vi "CRH3605KitList.vi"() -> ()   [LabVIEW 2012]
uses:
  <vilib>/addons/database/Connection.llb/DB Tools Open Connec (Path).vi
  Global1.vi
  <vilib>/Utility/file.llb/Read From Spreadsheet File (string).vi
  <vilib>/addons/database/NI_Database_API.lvlib
panel:
  out "error out":errorcluster
  in  "Cluster":T1
  out "String":string
  out "date/time string":string
  out "path":path
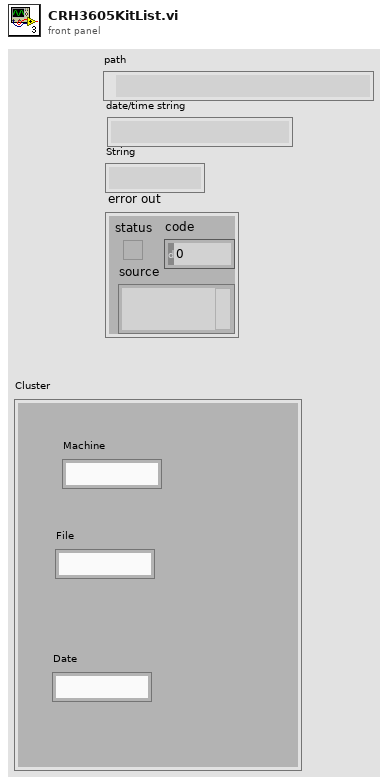
[diagram p1: front panel]
types:
  T1 = cluster{"Machine":string, "File":string, "Date":string}
  T2 = typedef "NI_Database_API.lvlib/Conn ObjectReference.ctl" = refnum<k1>
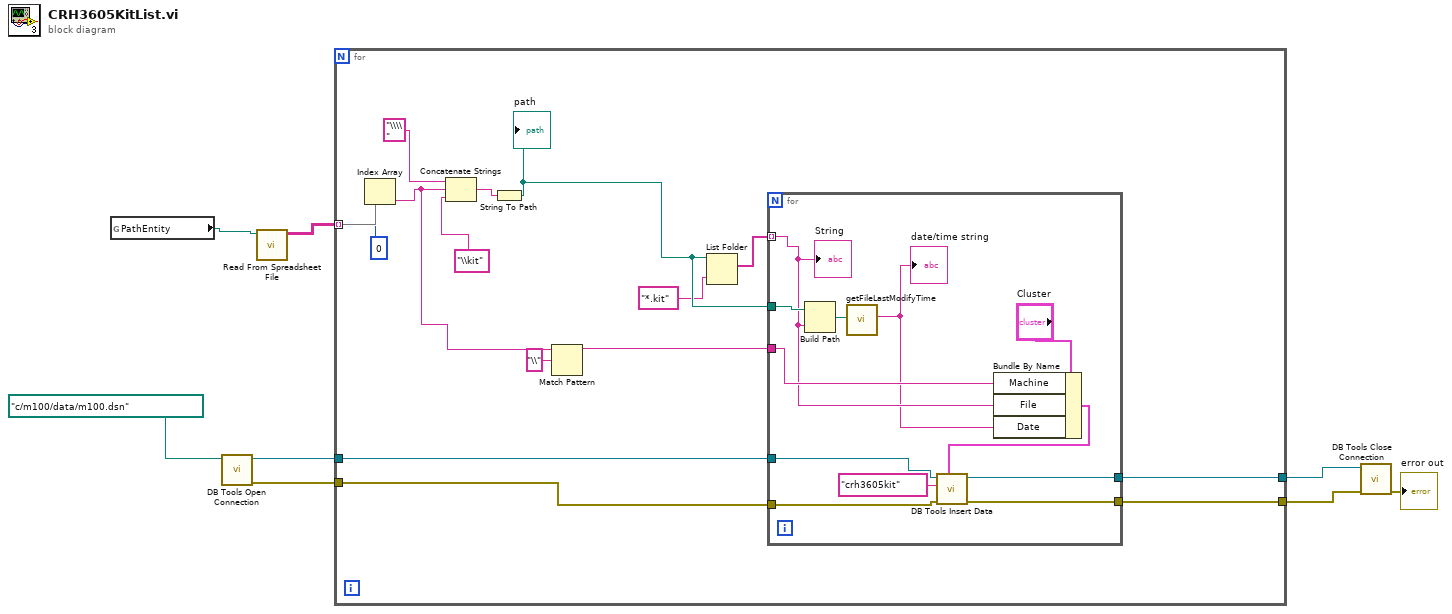
[diagram p0: block diagram]
diagram:
  n1 = global read "Global1.vi" "PathEntity"() -> (w8:path)
  n2 = call-poly <vilib>:"DB Tools Open Connection.vi"("connection information"=path "c:/m100/data/m100.dsn") -> ("error out"=w4:errorcluster, "connection reference"=w5:T2)  [unwired: 7 in]
  n3 = call-poly <vilib>:"Read From Spreadsheet File.vi"("file path (dialog if empty)"=w8) -> ("all rows"=w7:string[][])  [unwired: 6 in, 4 out]
  n4 = for {
    tunnel: w7 -> [w21] mode=indexing
    tunnel: w5 -> [w12]
    tunnel: w4 -> [w11]
    tunnel: [w10] -> w3
    tunnel: [w9] -> w2
    n5 = Index Array(array=w21, index=0) -> (element=w15:string)
    n6 = Concatenate Strings("\\\\" ("string"), w15, "\\kit") -> (w22:string)
    n7 = String To Path(string=w22) -> (path=w18:path)
    "path" <- w18
    n8 = Match Pattern(string=w15, regular expression="\\") -> (before substring=w13:string)  [unwired: 1 in, 3 out]
    n9 = List Folder(path=w18, pattern="*.kit") -> (filenames=w16:string[])  [unwired: 2 in, 3 out]
    n10 = for {
      tunnel: w18 -> [w35]
      tunnel: w16 -> [w31] mode=indexing
      tunnel: w13 -> [w32]
      tunnel: w12 -> [w29]
      tunnel: w11 -> [w28]
      tunnel: [w27] -> w10
      tunnel: [w26] -> w9
      n11 = Build Path(base path=w35, name or relative path=w31) -> (appended path=w34:path)
      n12 = call "getFileLastModifyTime.vi"("path"=w34) -> ("date/time string"=w30:string)  [unwired: 10 in]
      "date/time string" <- w30
      n13 = Bundle By Name(cluster="Cluster", "Machine"=w32, "File"=w31, "Date"=w30) -> (w24:T1)
      n14 = call <vilib>:"DB Tools Insert Data.vi"("data"=w24, "error in (no error)"=w28, "table"="crh3605kit", "connection reference"=w29) -> ("error out"=w26:errorcluster, "connection reference out"=w27:T2)  [unwired: 6 in]
      "String" <- w31
    }
  }
  n15 = call <vilib>:"DB Tools Close Connection.vi"("error in (no error)"=w2, "connection reference"=w3) -> ("error out"=→"error out":errorcluster)  [unwired: 5 in]
